vi "Find Closest Points.vi"(2 "Tag.lvclass":refnum<class "Tag.lvclass">, 3 "Intersection coordinates":dbl[][](array[numeric])) -> (0 "CenterOfGravityY":dbl, 1 "CenterOfGravityX":dbl)   [LabVIEW 2014, in "Position.lvclass"]
uses:
  Position.lvclass
  Tag.lvclass
panel:
  in  "Boolean":bool=TRUE
  out "size(s)":i32
  # "This VI finds the estimated position of the tag on the XY plane.\nThe input is the coordinates of the intersections."
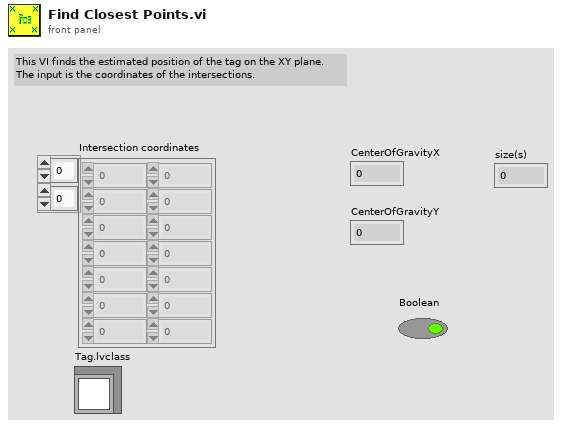
[diagram p1: front panel]
types:
  T1 = cluster{"X1":dbl, "Y1":dbl, "X2":dbl, "Y2":dbl, "Distance":dbl}[]
  T2 = cluster{"Numeric":dbl, "Numeric":dbl, "Numeric":dbl, "Numeric":dbl, "Distance":dbl}[]
  T3 = cluster{"Numeric":dbl, "Numeric":dbl, "Numeric":dbl, "Numeric":dbl, "Distance":dbl}
  T4 = cluster{"Numeric":dbl, "Numeric":dbl, "Numeric":dbl, "Numeric":dbl, "element":dbl}
  T5 = cluster{"Distance":dbl, cluster{"X1":dbl, "Y1":dbl, "X2":dbl, "Y2":dbl, "Distance":dbl}}
  T6 = cluster{"Distance":dbl, cluster{"X1":dbl, "Y1":dbl, "X2":dbl, "Y2":dbl, "Distance":dbl}}[]
  T7 = cluster{"X1":dbl, "Y1":dbl, "X2":dbl, "Y2":dbl, "Distance":dbl}
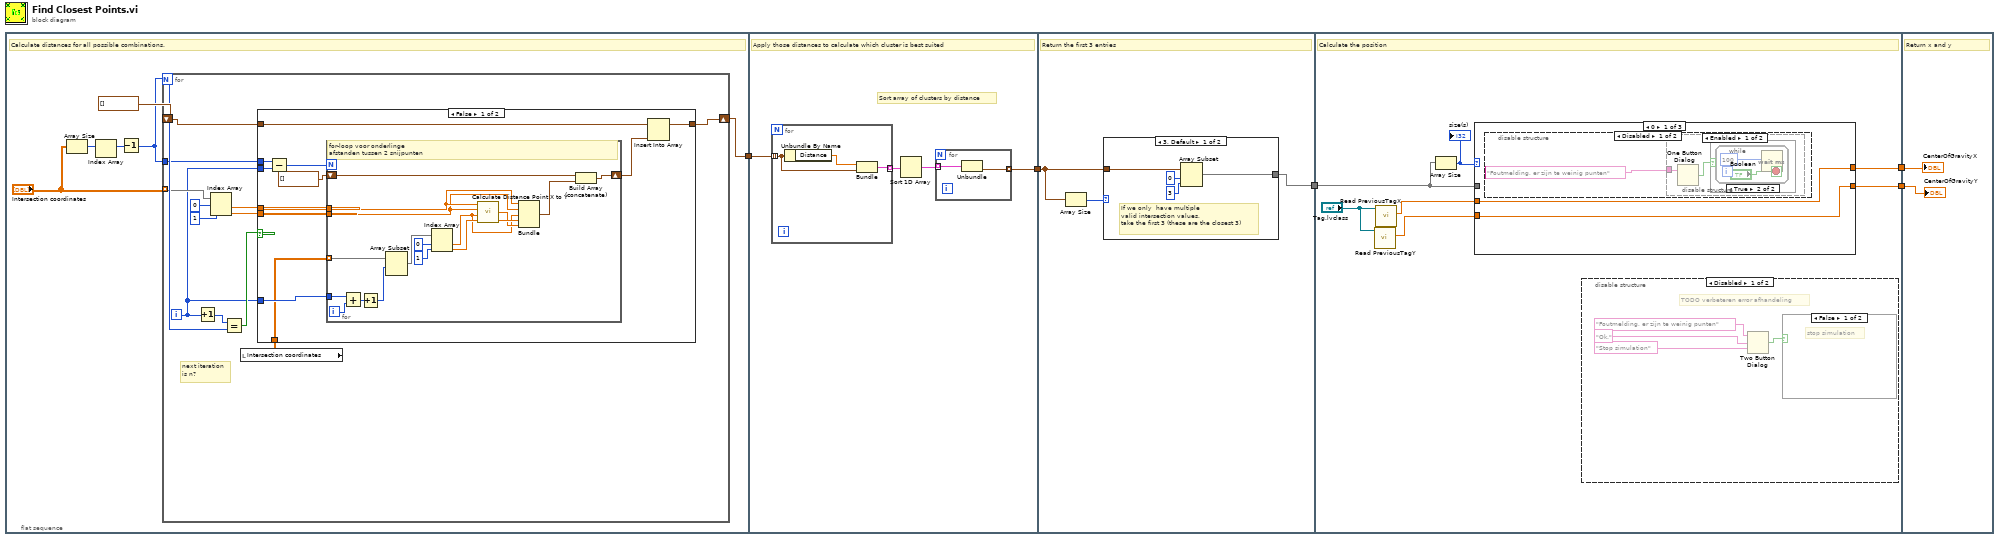
[diagram p0: block diagram]
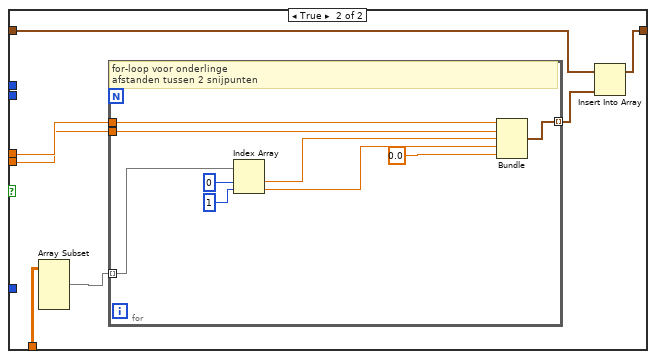
[diagram p2: hidden frame]
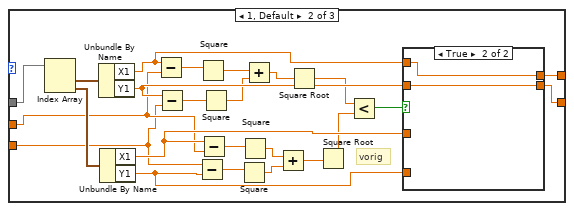
[diagram p9: hidden frame]
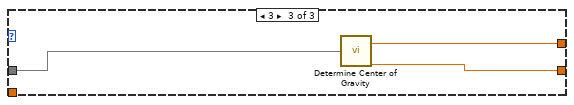
[diagram p11: hidden frame]
diagram:
  n1 = flat-sequence {
    tunnel: [w10] -> w5
    tunnel: w5 -> [w71]
    tunnel: [w68] -> w4
    tunnel: w4 -> [w79]
    tunnel: [w78] -> w1
    tunnel: [w91] -> w3
    tunnel: [w90] -> w2
    tunnel: w1 -> [w88]
    tunnel: w3 -> [w135]
    tunnel: w2 -> [w134]
    frame #0 {
      # "Calculate distances for all possible combinations."
      n2 = Array Size(array="Intersection coordinates") -> (size(s)=w8:i32[])
      n3 = Index Array(array=w8) -> (element=w7:i32)  [unwired: 1 in]
      n4 = Decrement(x=w7) -> (x-1=w6:i32)
      n5 = for {
        N: w6 -> [w20]
        tunnel: "Intersection coordinates" -> [w14] mode=indexing
        shift-right: [w15] -> w10
        shift-left: T1 [] -> [w16]
        tunnel: w6 -> [w13]
        i -> [w12]
        # "next iteration\nis n?"
        n6 = Increment(x=w12) -> (x+1=w19:i32)
        n7 = Index Array "Index Array"(array=w14, index #1=0 ("index"), index #2=1 ("index")) -> (element #1=w24:dbl, element #2=w23:dbl)
        n8 = Equal?(x=w19, y=w20) -> (x = y?=w17:bool)
        n9 = local read "Intersection coordinates"() -> (w18:dbl[][])
        n10 = case shown="False" w17 {
          tunnel: w24 -> [w35 w58]
          tunnel: w23 -> [w34 w57]
          tunnel: w18 -> [w28 w54]
          tunnel: w16 -> [w32 w53]
          tunnel: [w31 w52] -> w15
          tunnel: w12 -> [w30 _]
          tunnel: w13 -> [w26 _]
          tunnel: w12 -> [w25 _]
          frame False {
            n11 = Subtract(x=w26, y=w25) -> (x-y=w27:i32)
            n12 = for {
              N: w27 -> [_]
              tunnel: w35 -> [w51]
              tunnel: w34 -> [w50]
              tunnel: w30 -> [w46]
              shift-right: [w48] -> w33
              shift-left: T2 [] -> [w49]
              tunnel: w28 -> [w44] mode=indexing
              i -> [w47]
              # "for-loop voor onderlinge \nafstanden tussen 2 snijpunten"
              n13 = Add(x=w46, y=w47) -> (x+y=w45:i32)
              n14 = Increment(x=w45) -> (x+1=w43:i32)
              n15 = Array Subset(array=w44, index=w43) -> (w42:dbl[])  [unwired: 1 in]
              n16 = Index Array(array=w42, index #1=0 ("index"), index #2=1 ("index")) -> (element #1=w38:dbl, element #2=w40:dbl)
              n17 = call "Calculate Distance Point X to Y.vi"("Y 2"=w40, "X 2"=w38, "Y 1"=w50, "X 1"=w51) -> ("Distance"=w39:dbl)
              n18 = Bundle("Numeric"=w51, "Numeric"=w50, "Numeric"=w38, "Numeric"=w40, "Distance"=w39) -> (w36:T3)  [unwired: 1 in]
              n19 = Build Array (concatenate)(w49, w36) -> (w48:T2)
            }
            n20 = Insert Into Array(array=w32, new element=w33) -> (w31:T1)  [unwired: 1 in]
          }
          frame True {
            n21 = Array Subset(array=w54) -> (w55:dbl[][])  [unwired: 4 in]
            n22 = for {
              tunnel: w55 -> [w60] mode=indexing
              tunnel: w58 -> [w62]
              tunnel: w57 -> [w61]
              tunnel: [w64] -> w56 mode=indexing
              # "for-loop voor onderlinge \nafstanden tussen 2 snijpunten"
              n23 = Index Array(array=w60, index #1=0 ("index"), index #2=1 ("index")) -> (element #1=w65:dbl, element #2=w66:dbl)
              n24 = Bundle("Numeric"=w62, "Numeric"=w61, "Numeric"=w65, "Numeric"=w66, "element"=0.0) -> (w64:T4)  [unwired: 1 in]
            }
            n25 = Insert Into Array(array=w53, new element=w56) -> (w52:T1)  [unwired: 1 in]
          }
        }
      }
    }
    frame #1 {
      # "Sort array of clusters by distance"
      # "Apply those distances to calculate which cluster is best suited"
      n26 = for {
        tunnel: w71 -> [w76] mode=indexing
        tunnel: [w75] -> w70 mode=indexing
        n27 = Unbundle By Name(w76) -> ("Distance"=w74:dbl)
        n28 = Bundle("Distance"=w74, w76) -> (w75:T5)  [unwired: 1 in]
      }
      n29 = Sort 1D Array(array=w70) -> (sorted array=w69:T6)
      n30 = for {
        tunnel: w69 -> [w73] mode=indexing
        tunnel: [w72] -> w68 mode=indexing
        n31 = Unbundle(w73) -> (w72:T7)  [unwired: 1 out]
      }
    }
    frame #2 {
      # "Return the first 3 entries"
      n32 = Array Size(array=w79) -> (size(s)=w77:i32)
      n33 = case shown="3, Default" w77 {
        tunnel: w79 -> [w81 w84]
        tunnel: [w80 w84] -> w78
        frame 3, Default {
          # "If we only  have multiple \nvalid intersection values,\ntake the first 3 (these are the closest 3)"
          n34 = Array Subset(array=w81, index=0, length=3) -> (w80:T1)
        }
        frame 0, 1 {
          # "If we only have 2 valid intersection values"
        }
      }
    }
    frame #3 {
      # "Calculate the position"
      n35 = call-dynamic "Read PreviousTagY.vi"("Tag in"="Tag.lvclass") -> ("PreviousTagY"=w85:dbl)  [unwired: 8 in, 2 out]
      n36 = call-dynamic "Read PreviousTagX.vi"("Tag in"="Tag.lvclass") -> ("PreviousTagX"=w86:dbl)  [unwired: 8 in, 2 out]
      n37 = Array Size(array=w88) -> (size(s)=w89:i32)
      "size(s)" <- w89
      n38 = case shown="0" w89 {
        tunnel: [w97 w121 w133] -> w91
        tunnel: [w96 w120 w132] -> w90
        tunnel: w88 -> [_ w126 w131]
        tunnel: w86 -> [w97 w104 _]
        tunnel: w85 -> [w96 w103 _]
        frame 0 {
          n39 = disable-structure shown="Disabled" {
            frame Disabled {
              n40 = disable-structure shown="Enabled" {
                disable-tunnel: "Foutmelding, er zijn te weinig punten" ("message") -> [w100 _]
                frame Enabled {
                  n41 = One Button Dialog(message=w100) -> (true=w99:bool)  [unwired: 1 in]
                  n42 = case shown="True" w99 {
                    frame False {
                    }
                    frame True {
                      n43 = while {
                        stop <- "Boolean" stop-if-true
                        n44 = Wait (ms)(milliseconds to wait=u32 100) -> ()  [unwired: 1 out]
                      }
                    }
                  }
                }
                frame Disabled {
                }
              }
            }
            frame Enabled {
            }
          }
        }
        frame 1, Default {
          # "vorig"
          n45 = Index Array(array=w126) -> (element #1=w125:T7, element #2=w124:T7)  [unwired: 2 in]
          n46 = Unbundle By Name(w125) -> ("X1"=w122:dbl, "Y1"=w119:dbl)
          n47 = Unbundle By Name(w124) -> ("X1"=w118:dbl, "Y1"=w117:dbl)
          n48 = Subtract(x=w122, y=w104) -> (x-y=w116:dbl)
          n49 = Subtract(x=w119, y=w103) -> (x-y=w115:dbl)
          n50 = Subtract(x=w103, y=w117) -> (x-y=w113:dbl)
          n51 = Square(x=w116) -> (x^2=w112:dbl)
          n52 = Subtract(x=w118, y=w104) -> (x-y=w114:dbl)
          n53 = Square(x=w115) -> (x^2=w111:dbl)
          n54 = Square(x=w113) -> (x^2=w109:dbl)
          n55 = Square(x=w114) -> (x^2=w110:dbl)
          n56 = Add(x=w112, y=w111) -> (x+y=w108:dbl)
          n57 = Add(x=w110, y=w109) -> (x+y=w107:dbl)
          n58 = Square Root(x=w108) -> (sqrt(x)=w105:dbl)
          n59 = Square Root(x=w107) -> (sqrt(x)=w106:dbl)
          n60 = Less?(x=w105, y=w106) -> (x < y?=w123:bool)
          n61 = case shown="True" w123 {
            tunnel: w122 -> [_ w130]
            tunnel: [w128 w130] -> w121
            tunnel: w119 -> [_ w129]
            tunnel: [w127 w129] -> w120
            tunnel: w118 -> [w128 _]
            tunnel: w117 -> [w127 _]
            frame False {
            }
            frame True {
            }
          }
        }
        frame 3 {
          n62 = call "Determine Center of Gravity.vi"("Input Intersections"=w131) -> ("CenterOfGravity X"=w133:dbl, "CenterOfGravity Y"=w132:dbl)
        }
      }
      n63 = disable-structure shown="Disabled" {
        frame Disabled {
          # "TODO verbeteren error afhandeling"
          n64 = Two Button Dialog(message="Foutmelding, er zijn te weinig punten", 1:"Stop simulation" ("F button name (\"Cancel\")"), 2:"Ok." ("T button name (\"OK\")")) -> (T button?=w92:bool)
          n65 = case shown="False" w92 {
            frame False {
              # "stop simulation"
            }
            frame True {
            }
          }
        }
        frame Enabled {
        }
      }
    }
    frame #4 {
      # "Return x and y"
      "CenterOfGravityX" <- w135
      "CenterOfGravityY" <- w134
    }
  }
